vi "UnInstall and instal.vi"   [LabVIEW 2014]
panel:
  # "Unistal and instal new version"
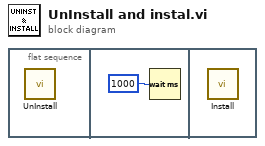
[diagram p0: block diagram]
diagram:
  n1 = flat-sequence {
    frame #0 {
      n2 = call "UnInstall.vi"() -> ()  [unwired: 12 in]
    }
    frame #1 {
      n3 = Wait (ms)(milliseconds to wait=u32 1000) -> ()  [unwired: 1 out]
    }
    frame #2 {
      n4 = call "Install.vi"() -> ()  [unwired: 12 in]
    }
  }
